vi "criticity safety.vi"() -> ()   [LabVIEW 2020]
uses:
  <vilib>/Utility/miscctls.llb/LVAnnotationListTypeDef.ctl
  <vilib>/Analysis/baseanly.llb/Mean (DBL).vi
  global/SettingVariable.vi
  <userlib>/_OpenG.lib/array/array.llb/Empty 2D Array (DBL)__ogtk.vi
  <vilib>/express/express arith-compare/Formula/XNode/ExpressFormulaBlockNode.xnode
  <vilib>/Analysis/NI_AALBase.lvlib
  <vilib>/Analysis/NI_AALPro.lvlib
panel:
  out "历史波形图":cluster{dbl, dbl, dbl[][]}(graph)
  out "左选标时刻":timestamp caption="左选标时刻：" format="%<%.2X %x>T"
  out "数据点数":i32 caption="选中的数据点数："
  out "通量通道均值":dbl
  out "临界途径均值":dbl
  in  "临界途径":u16(ring) caption="临界途径：" items=["棒位D"]
  in  "通量通道":u16(ring) caption="通量通道：" items=["电压8", "电流1", "电流2"]
  out "采样间隔":dbl
  out "开始时间":timestamp
  in  "在线数据":bool
  in  "打开文件":bool
  out "记录表":string[][](table) caption="计算结果记录表"
  out "临界外推趋势图":cluster{dbl[], dbl[]}[](graph) caption="XY Graph - Dark"
  in  "保存表格":bool
  in  "添加记录":bool
  out "提示信息":string="载入数据后，拖动波形图中的游标选取数据添加记录。"
  out "文件信息":string
  # "坐标轴与图例"
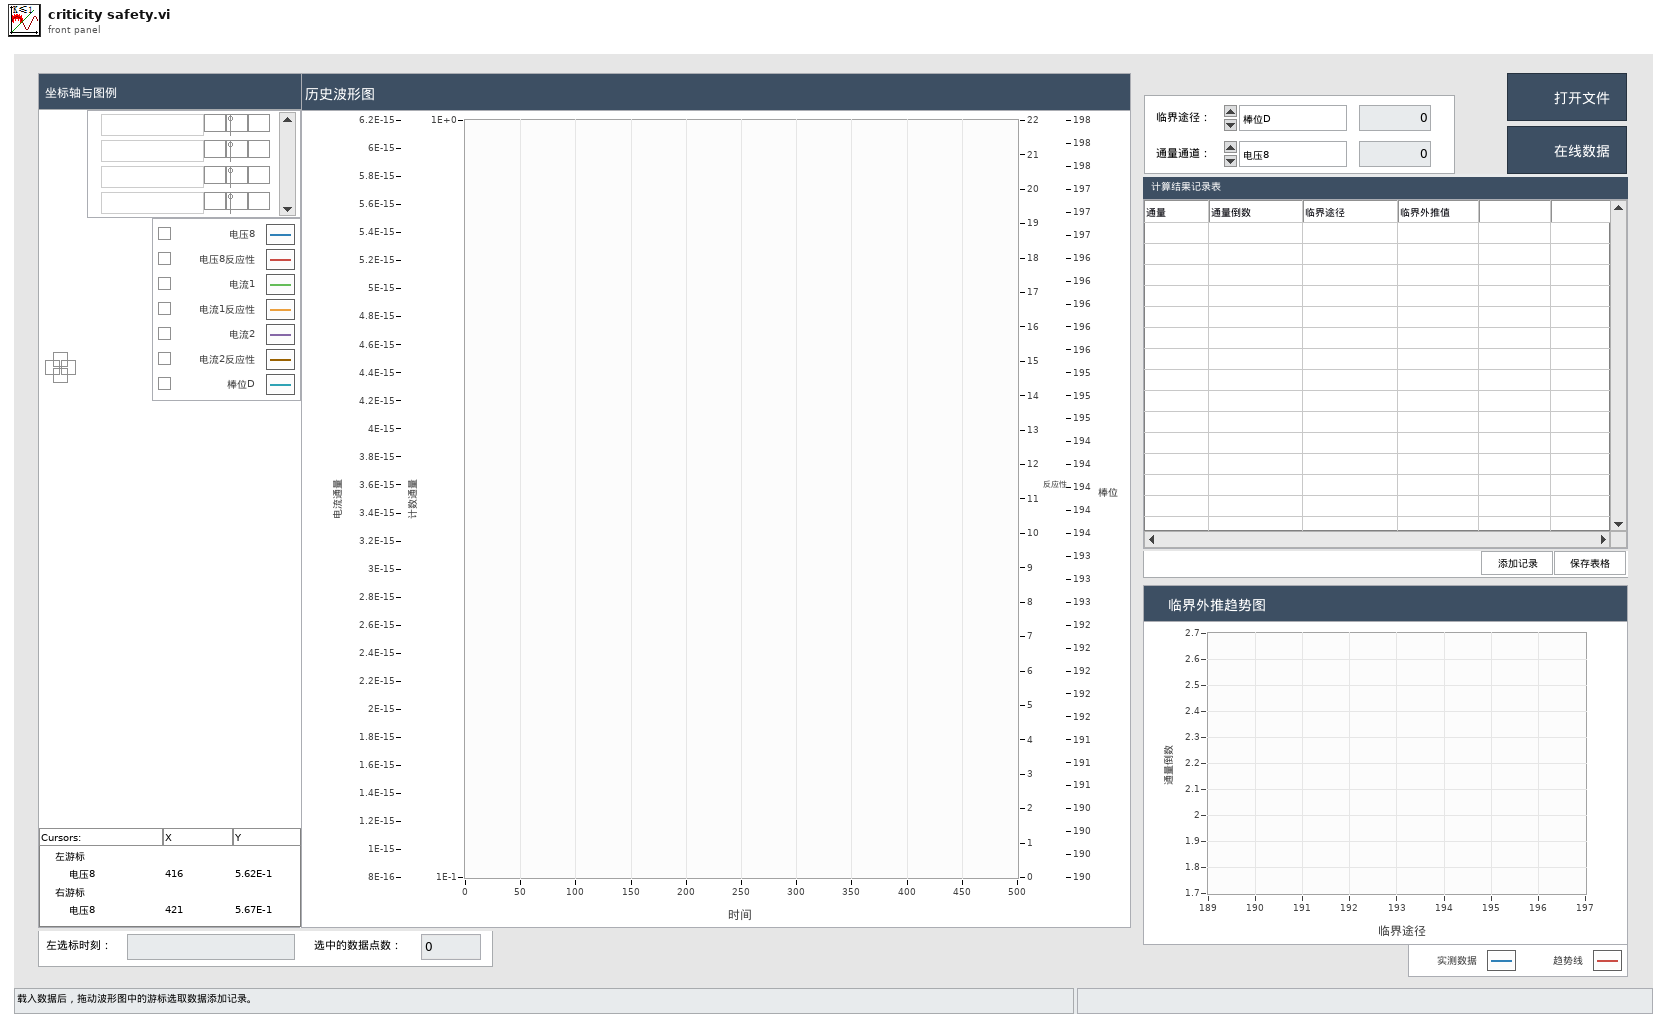
[diagram p1: front panel]
types:
  T1 = typedef "LVAnnotationListTypeDef.ctl" = cluster{"Name":string, "Color":u32, "Style":u8, "Point Style":u8, "Name Visible":bool, "Allow Drag":bool, "Annotation Mode":u32, "Plot":i32, "Index":i32, "Position":cluster{"X":dbl, "Y":dbl}, "X Scale":u32, "Y Scale":u32, "Show Arrow":bool, "Lock Name":bool, "Plot Area":i32, "Label Offset":cluster{"X":dbl, "Y":dbl}}[]
  T2 = cluster{"Name":string, "Color":u32, "Style":u8, "Point Style":u8, "Name Visible":bool, "Allow Drag":bool, "Annotation Mode":u32, "Plot":i32, "Index":i32, "Position":cluster{"X":dbl, "Y":dbl}, "X Scale":u32, "Y Scale":u32, "Show Arrow":bool, "Lock Name":bool, "Plot Area":i32, "Label Offset":cluster{"X":dbl, "Y":dbl}}
  T3 = enum16{"open", "replace", "create", "open or create", "replace or create", "replace or create with confirmation"}
  T4 = typedef "LVCursorListTypeDef.ctl" = cluster{"Name":string, "Color":u32, "Style":u8, "Point Style":u8, "Name Visible":bool, "Allow Drag":bool, "Cursor Mode":u32, "Plot":i32, "Index":i32, "Position":cluster{"X":dbl, "Y":dbl}, "X Scale":u32, "Y Scale":u32, "Watch Plots":i32[], "Watch All Plots":bool, "Plot Area":i32, "Label Offset":cluster{"X":dbl, "Y":dbl}}[]
  T5 = cluster{"Name":string, "Color":u32, "Style":u8, "Point Style":u8, "Name Visible":bool, "Allow Drag":bool, "Cursor Mode":u32, "Plot":i32, "Index":i32, "Position":cluster{"X":dbl, "Y":dbl}, "X Scale":u32, "Y Scale":u32, "Watch Plots":i32[], "Watch All Plots":bool, "Plot Area":i32, "Label Offset":cluster{"X":dbl, "Y":dbl}}
  T6 = enum32{"invalid app kind", "Development System", "Run Time System", "Student Edition", "Embedded LabVIEW", "Evaluation", "Custom"}
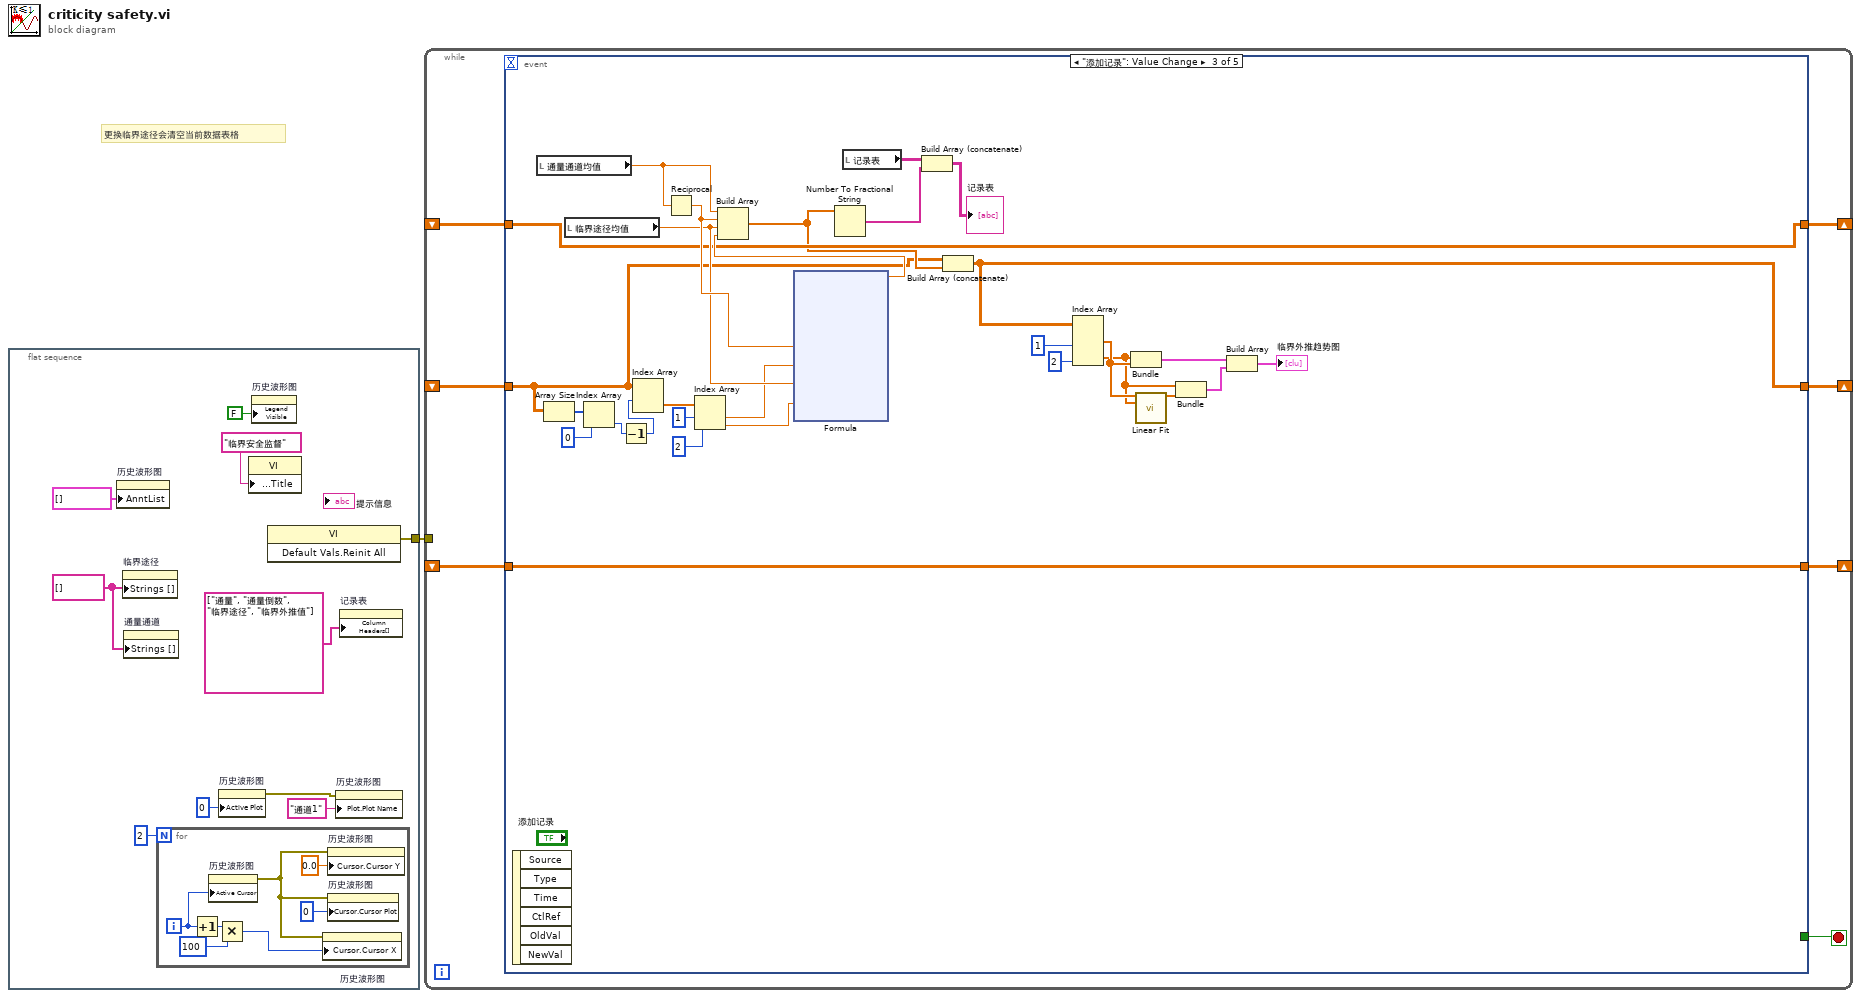
[diagram p0: block diagram]
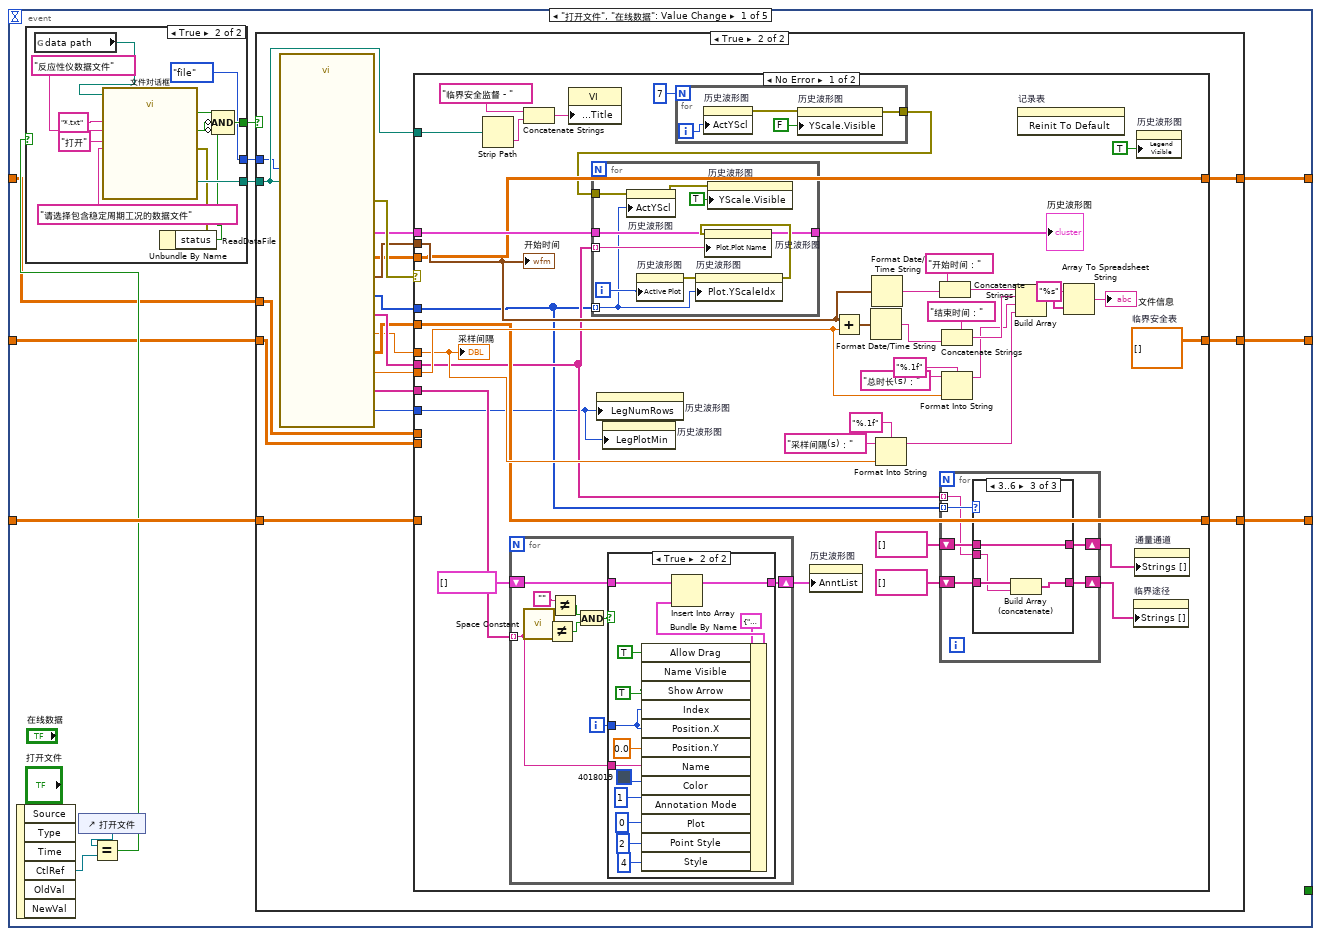
[diagram p2: hidden frame]
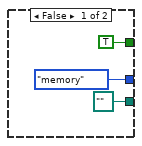
[diagram p3: hidden frame]
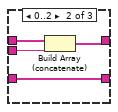
[diagram p6: hidden frame]
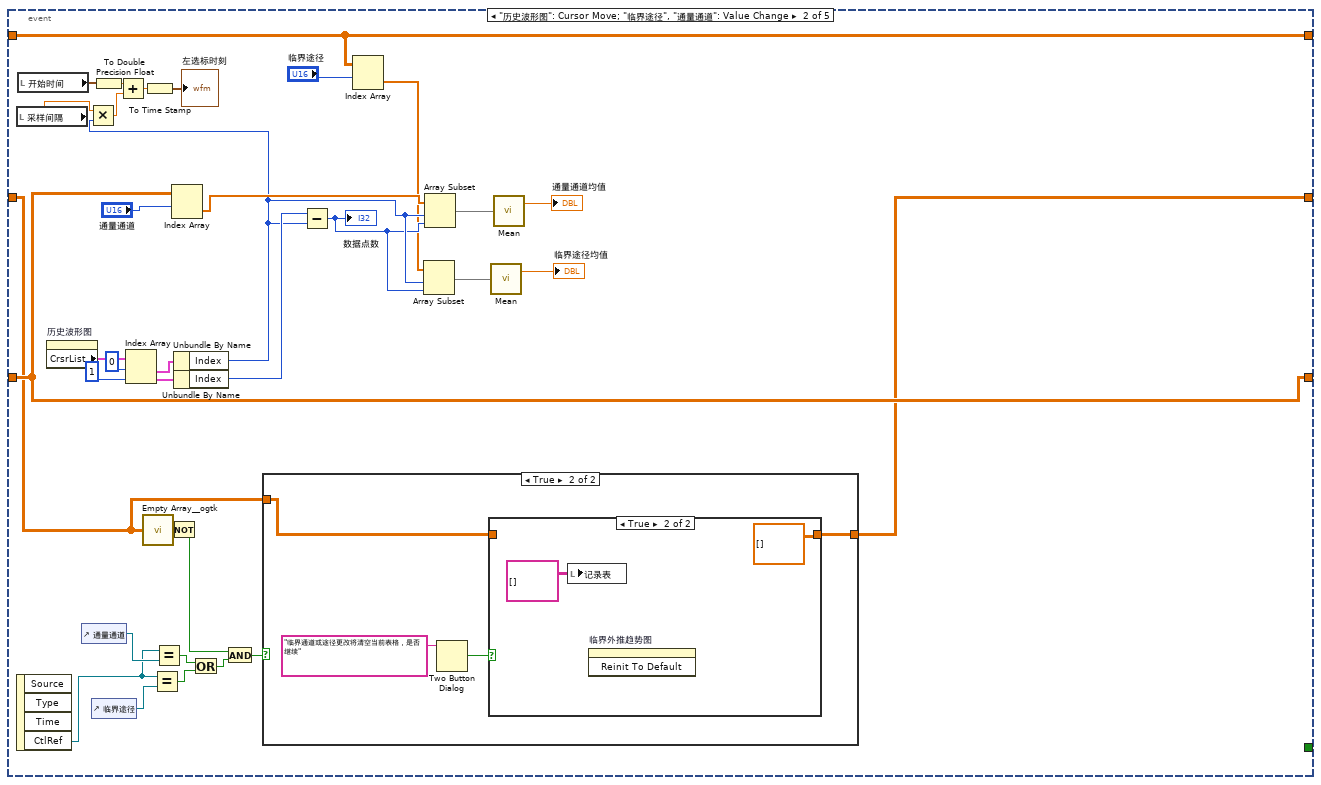
[diagram p9: hidden frame]
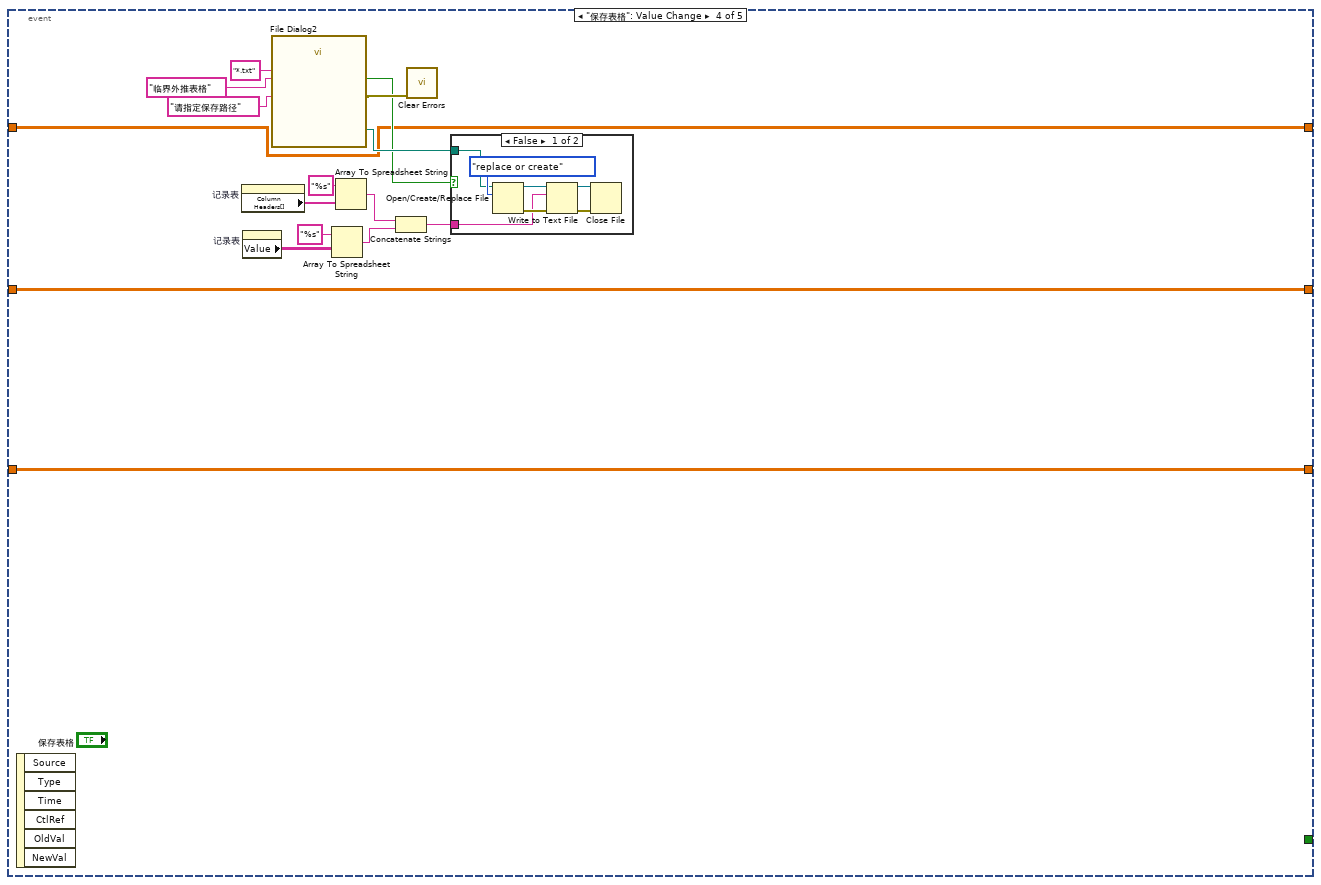
[diagram p12: hidden frame]
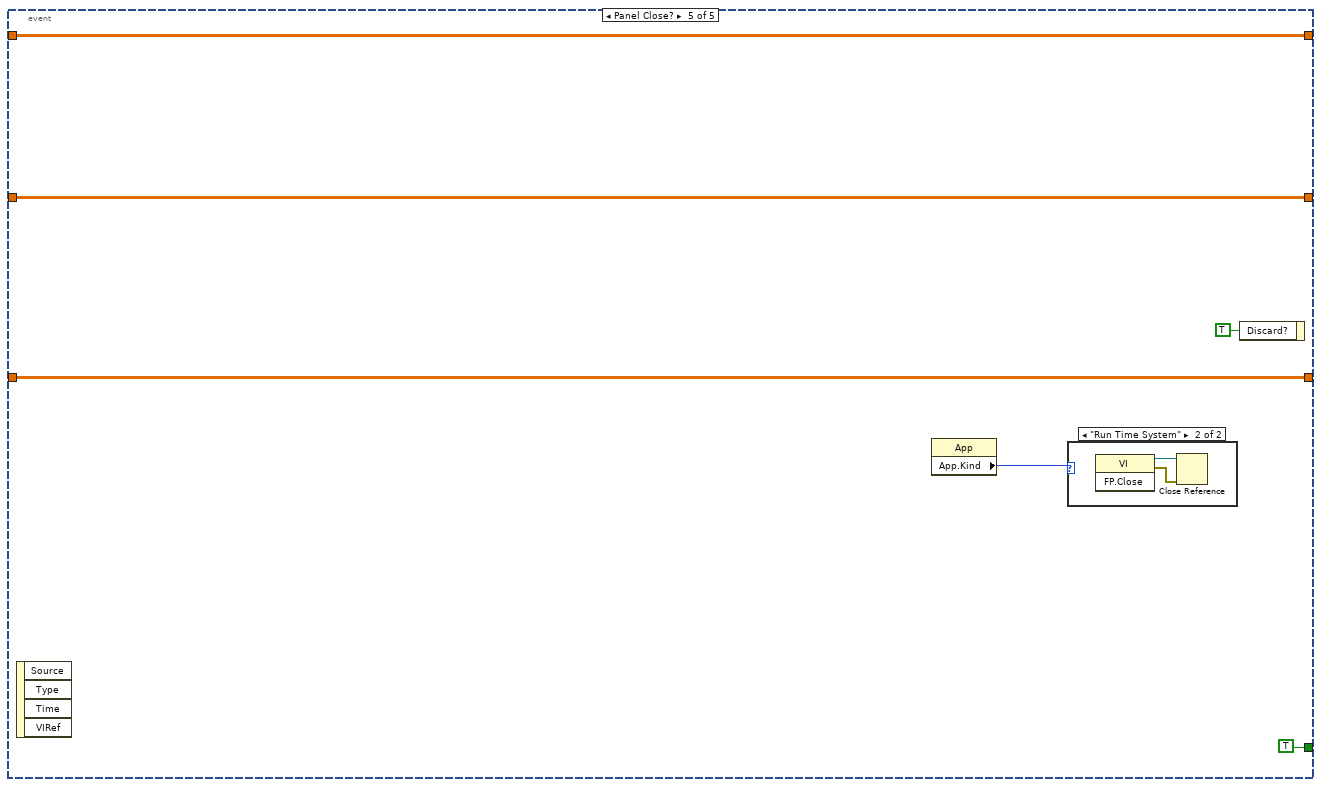
[diagram p14: hidden frame]
diagram:
  # "更换临界途径会清空当前数据表格"
  n1 = flat-sequence {
    tunnel: [w7] -> w1
    frame #0 {
      w2 = string[] [] ("Strings []")
      n2 = property on="历史波形图" class="WFGraph (strict)"("AnntList"=T1 [] ("Annotation List")) -> ()  [unwired: 2 in, 2 out]
      n3 = property on="临界途径" class="Ring (strict)"("Strings []"=w2) -> ()  [unwired: 2 in, 2 out]
      n4 = property on="通量通道" class="Ring (strict)"("Strings []"=w2) -> ()  [unwired: 2 in, 2 out]
      n5 = for {
        N: 2 -> [_]
        i -> [w16]
        n6 = Increment(x=w16) -> (x+1=w15:i32)
        n7 = property on="历史波形图" class="WFGraph (strict)"("Active Cursor"=w16) -> (error out=w12:errorcluster)  [unwired: 2 in, 1 out]
        n8 = Multiply(x=w15, y=100) -> (x*y=w13:i32)
        n9 = property on="历史波形图" class="WFGraph (strict)"(error in=w12, "Cursor.Cursor X"=w13) -> ()  [unwired: 1 in, 2 out]
        n10 = property on="历史波形图" class="WFGraph (strict)"(error in=w12, "Cursor.Cursor Y"=0.0 ("Cursor.Cursor Position:Cursor Y")) -> ()  [unwired: 1 in, 2 out]
        n11 = property on="历史波形图" class="WFGraph (strict)"(error in=w12, "Cursor.Cursor Plot"=0 ("Cursor.Cursor Index")) -> ()  [unwired: 1 in, 2 out]
      }
      n12 = property on="历史波形图" class="WFGraph (strict)"("Active Plot"=u32 0) -> (error out=w9:errorcluster)  [unwired: 2 in, 1 out]
      n13 = property class="VI"("Front Panel.Title"="临界安全监督" ("Front Panel Window:Title")) -> ()  [unwired: 2 in, 2 out]
      n14 = property on="历史波形图" class="WFGraph (strict)"("Legend Visible"=FALSE ("Legend:Visible")) -> ()  [unwired: 2 in, 2 out]
      n15 = invoke class="VI" method="Default Vals.Reinit All"() -> (error out=w7:errorcluster)  [unwired: 3 in, 2 out]
      n16 = property on="历史波形图" class="WFGraph (strict)"(error in=w9, "Plot.Plot Name"="通道1") -> ()  [unwired: 1 in, 2 out]
      n17 = property on="记录表" class="Tbl (strict)"("Column Headers[]"=string[] ["通量", "通量倒数", "临界途径", "临界外推值"] ("行首字符串[]")) -> ()  [unwired: 2 in, 2 out]
    }
  }
  n18 = while {
    shift-right: [w25] -> _
    shift-left: _ -> [w24]
    tunnel: w1 -> [_]
    shift-right: [w22] -> _
    shift-left: _ -> [w21]
    shift-right: [w19] -> _
    shift-left: _ -> [w20]
    stop <- w23 stop-if-true
    n19 = event shown="[2] \"添加记录\": Value Change" {
      selector: _ -> [_ _ _ _ _]
      dyn-events: _ -> [_ _ _ _ _]
      timeout: _ -> [_ _ _ _ _]
      tunnel: [w36 w184 w243 w273 w282] -> w25
      tunnel: w24 -> [w35 w184 w243 w273 w282]
      tunnel: [_ _ _ _ TRUE] -> w23
      tunnel: [w29 w183 w226 w259 w283] -> w22
      tunnel: w21 -> [w28 w183 w226 w259 w283]
      tunnel: w20 -> [w26 w173 w224 w258 w281]
      tunnel: [w27 w172 w223 w258 w281] -> w19
      event "打开文件", "在线数据": Value Change {
        n20 = event-data() -> ("CtlRef"=w33:refnum<vi>)  [unwired: 1 in, 5 out]
        n21 = control-ref of="打开文件"() -> (w32:refnum<vi>)
        n22 = Equal?(x=w32, y=w33) -> (x = y?=w31:bool)
        n23 = case shown="True" w31 {
          tunnel: [path "" ("selected path") w52] -> w37
          tunnel: [TRUE w43] -> w34
          tunnel: [enum16{"file", "memory"}."memory" ("source") enum16{"file", "memory"}."file" ("source")] -> w30
          frame False {
          }
          frame True {
            n24 = global read "SettingVariable.vi" "data path"() -> (w42:path)
            n25 = call "文件对话框"("start path"=w42, "prompt"="请选择包含稳定周期工况的数据文件", "button label"="打开", "pattern (all files)"="*.txt", "pattern label"="反应性仪数据文件") -> ("selected path"=w52:path, "exists"=w46:bool, "cancelled"=w45:bool, "error out"=w47:errorcluster)  [unwired: 7 in]
            n26 = Unbundle By Name(w47) -> ("status"=w44:bool)
            n27 = Compound Arithmetic op=AND(w46, invert w45, invert w44) -> (w43:bool)
          }
        }
        n28 = case shown="True" w34 {
          tunnel: w37 -> [_ w62]
          tunnel: [w55 w66] -> w36
          tunnel: w35 -> [w55 w65]
          tunnel: w30 -> [_ w61]
          tunnel: [w54 w59] -> w29
          tunnel: w28 -> [w54 w58]
          tunnel: [w53 w57] -> w27
          tunnel: w26 -> [w53 w56]
          frame False {
          }
          frame True {
            n29 = call "ReadDataFile.vi"("file path"=w62, "source"=w61) -> ("曲线对应标尺编号"=w69:i32[], "曲线名"=w68:string[], "通量数据"=w67:dbl[][], "时间间隔"=w64:dbl, "P2数据"=w60:dbl[][], "曲线数"=w71:i32, "开始时间"=w63:timestamp, "总时长(s)"=w72:dbl, "error out"=w74:errorcluster, "备注数组"=w70:string[], "波形簇"=w73:cluster{dbl, dbl, dbl[][]})  [unwired: 1 in, 2 out]
            n30 = case shown="No Error" w74 {
              tunnel: w73 -> [w87 _]
              tunnel: w72 -> [w106 _]
              tunnel: w71 -> [w75 _]
              tunnel: w70 -> [w113 _]
              tunnel: w69 -> [w78 _]
              tunnel: w68 -> [w83 _]
              tunnel: w67 -> [w84 _]
              tunnel: [w84 w171] -> w66
              tunnel: w65 -> [_ w171]
              tunnel: w64 -> [w104 _]
              tunnel: w63 -> [w111 _]
              tunnel: w62 -> [w90 _]
              tunnel: w60 -> [w86 _]
              tunnel: [w86 w170] -> w59
              tunnel: w58 -> [_ w170]
              tunnel: [w85 w169] -> w57
              tunnel: w56 -> [_ w169]
              frame No Error {
                w85 = dbl[][] []  # 临界安全表
                n31 = Strip Path(path=w90) -> (name=w91:string)  [unwired: 1 out]
                n32 = for {
                  tunnel: w113 -> [w148] mode=indexing
                  shift-right: [w150] -> w115
                  shift-left: T1 [] ("注释列表") -> [w151]
                  i -> [w152]
                  n33 = call <vilib>:"Space Constant.vi"() -> ("String"=w153:string)
                  n34 = Not Equal?(x=w153, y=w148) -> (x != y?=w146:bool)
                  n35 = Not Equal?(x="", y=w148) -> (x != y?=w147:bool)
                  n36 = And(x=w147, y=w146) -> (x .and. y?=w145:bool)
                  n37 = case shown="True" w145 {
                    tunnel: w148 -> [_ w163]
                    tunnel: w152 -> [_ w165]
                    tunnel: w151 -> [w154 w168]
                    tunnel: [w154 w167] -> w150
                    frame False {
                    }
                    frame True {
                      w166 = TRUE ("Show Arrow")
                      n38 = Bundle By Name(cluster=T2 {"Name"="", "Color"=0, "Style"=0, "Point Style"=0, "Name Visible"=FALSE, "Allow Drag"=FALSE, "Annotation Mode"=0, "Plot"=0, "Index"=0, "Position"={"X"=0.0, "Y"=0.0}, "X Scale"=0, "Y Scale"=0, "Show Arrow"=FALSE, "Lock Name"=FALSE, "Plot Area"=0, "Label Offset"={"X"=0.0, "Y"=0.0}} ("元素"), "Allow Drag"=TRUE, "Name Visible"=w166, "Show Arrow"=w166, "Index"=w165, "Position.X"=w165, "Position.Y"=0.0 ("Y"), "Name"=w163, "Color"=u32 4018019, "Annotation Mode"=u32 1, "Plot"=0, "Point Style"=u8 2, "Style"=u8 4) -> (w164:T2)
                      n39 = Insert Into Array(array=w168, new element=w164) -> (w167:T1)  [unwired: 1 in]
                    }
                  }
                }
                n40 = Concatenate Strings("临界安全监督 - " ("string"), w91) -> (w92:string)
                n41 = property class="VI"("Front Panel.Title"=w92) -> ()  [unwired: 2 in, 2 out]
                n42 = property on="历史波形图" class="WFGraph (strict)"("LegNumRows"=w75) -> ()  [unwired: 2 in, 2 out]
                n43 = property on="历史波形图" class="WFGraph (strict)"("LegPlotMin"=w75) -> ()  [unwired: 2 in, 2 out]
                n44 = for {
                  N: 7 -> [_]
                  tunnel: [w117] -> w76
                  i -> [w116]
                  n45 = property on="历史波形图" class="WFGraph (strict)"("ActYScl"=w116) -> (error out=w118:errorcluster)  [unwired: 2 in, 1 out]
                  n46 = property on="历史波形图" class="WFGraph (strict)"(error in=w118, "YScale.Visible"=FALSE ("Y Scale.Visible")) -> (error out=w117:errorcluster)  [unwired: 1 in, 1 out]
                }
                n47 = for {
                  tunnel: w78 -> [w139] mode=indexing
                  tunnel: w83 -> [w141] mode=indexing
                  tunnel: [w140] -> w88
                  tunnel: w87 -> [w140]
                  tunnel: w76 -> [w136]
                  i -> [w142]
                  n48 = property on="历史波形图" class="WFGraph (strict)"(error in=w136, "ActYScl"=w139) -> (error out=w137:errorcluster)  [unwired: 1 in, 1 out]
                  n49 = property on="历史波形图" class="WFGraph (strict)"("Active Plot"=w142) -> (error out=w144:errorcluster)  [unwired: 2 in, 1 out]
                  n50 = property on="历史波形图" class="WFGraph (strict)"(error in=w144, "Plot.YScaleIdx"=w139) -> (error out=w143:errorcluster)  [unwired: 1 in, 1 out]
                  n51 = property on="历史波形图" class="WFGraph (strict)"(error in=w143, "Plot.Plot Name"=w141) -> ()  [unwired: 1 in, 2 out]
                  n52 = property on="历史波形图" class="WFGraph (strict)"(error in=w137, "YScale.Visible"=TRUE ("Y Scale.Visible")) -> ()  [unwired: 1 in, 2 out]
                }
                "历史波形图" <- w88
                n53 = property on="历史波形图" class="WFGraph (strict)"("AnntList"=w115) -> ()  [unwired: 2 in, 2 out]
                n54 = Add(x=w111, y=w106) -> (x+y=w112:timestamp)
                n55 = Format Date/Time String(seconds (now)=w112) -> (date/time string=w107:string)  [unwired: 2 in]
                n56 = Format Date/Time String(seconds (now)=w111) -> (date/time string=w109:string)  [unwired: 2 in]
                n57 = Format Into String(format string="%.1f", initial string="采样间隔(s)：", w104) -> (resulting string=w97:string)  [unwired: 1 in, 1 out]
                n58 = Concatenate Strings("开始时间：" ("string"), w109) -> (w102:string)
                n59 = for {
                  tunnel: w83 -> [w120] mode=indexing
                  shift-right: [w121] -> w80
                  shift-left: string[] [] ("Strings []") -> [w122]
                  shift-right: [w123] -> w79
                  shift-left: string[] [] ("Strings []") -> [w124]
                  tunnel: w78 -> [w125] mode=indexing
                  n60 = case shown="3..6" w125 {
                    tunnel: w124 -> [w127 w131 w135]
                    tunnel: [w127 w130 w135] -> w123
                    tunnel: w122 -> [w126 w128 w134]
                    tunnel: [w126 w128 w132] -> w121
                    tunnel: w120 -> [_ w129 w133]
                    frame 7, Default {
                    }
                    frame 0..2 {
                      n61 = Build Array (concatenate)(w131, w129) -> (w130:string[])
                    }
                    frame 3..6 {
                      n62 = Build Array (concatenate)(w134, w133) -> (w132:string[])
                    }
                  }
                }
                n63 = Concatenate Strings("结束时间：" ("string"), w107) -> (w99:string)
                n64 = Format Into String(format string="%.1f", initial string="总时长(s)：", w106) -> (resulting string=w98:string)  [unwired: 1 in, 1 out]
                n65 = Build Array(w102, w99, w98, w97) -> (w101:string[])
                n66 = invoke on="记录表" class="Tbl (strict)" method="Reinit To Default"() -> ()  [unwired: 3 in, 3 out]
                n67 = Array To Spreadsheet String(array=w101, 3:"%s" ("format string")) -> (spreadsheet string=→"文件信息":string)  [unwired: 1 in]
                n68 = property on="临界途径" class="Ring (strict)"("Strings []"=w80) -> ()  [unwired: 2 in, 2 out]
                n69 = property on="通量通道" class="Ring (strict)"("Strings []"=w79) -> ()  [unwired: 2 in, 2 out]
                n70 = property on="历史波形图" class="WFGraph (strict)"("Legend Visible"=TRUE ("Legend:Visible")) -> ()  [unwired: 2 in, 2 out]
                "开始时间" <- w111
                "采样间隔" <- w104
              }
              frame Error {
              }
            }
          }
        }
      }
      event "历史波形图": Cursor Move; "临界途径", "通量通道": Value Change {
        n71 = local read "采样间隔"() -> (w195:dbl)
        n72 = event-data() -> ("CtlRef"=w180:refnum<vi>)  [unwired: 1 in, 3 out]
        n73 = local read "开始时间"() -> (w196:timestamp)
        n74 = property on="历史波形图" class="WFGraph (strict)"() -> ("CrsrList"=w202:T4)  [unwired: 2 in, 2 out]
        n75 = control-ref of="通量通道"() -> (w181:refnum<vi>)
        n76 = control-ref of="临界途径"() -> (w182:refnum<vi>)
        n77 = To Double Precision Float(number=w196) -> (double precision float=w201:dbl)
        n78 = Index Array(array=w202, index #1=0 ("index"), index #2=1 ("index")) -> (element #1=w204:T5, element #2=w206:T5)
        n79 = call-poly <userlib>:"Empty Array__ogtk.vi"("Array"=w173) -> ("Empty Array?"=w177:bool)  [unwired: 8 in]
        n80 = Equal?(x=w180, y=w182) -> (x = y?=w178:bool)
        n81 = Equal?(x=w180, y=w181) -> (x = y?=w179:bool)
        n82 = Not(x=w177) -> (.not. x?=w176:bool)
        n83 = Index Array(array=w184, index (row)="通量通道") -> (element=w192:dbl[])  [unwired: 1 in]
        n84 = Unbundle By Name(w204) -> ("Index"=w188:i32)
        n85 = Multiply(x=w195, y=w188) -> (x*y=w198:dbl)
        n86 = Add(x=w201, y=w198) -> (x+y=w200:dbl)
        n87 = To Time Stamp(1:w200) -> (0:→"左选标时刻":timestamp)
        n88 = Unbundle By Name(w206) -> ("Index"=w197:i32)
        n89 = Or(x=w179, y=w178) -> (x .or. y?=w175:bool)
        n90 = And(x=w176, y=w175) -> (x .and. y?=w174:bool)
        n91 = case shown="True" w174 {
          tunnel: w173 -> [w207 w209]
          tunnel: [w207 w208] -> w172
          frame False {
          }
          frame True {
            n92 = Two Button Dialog(message="临界通道或途径更改将清空当前表格，是否继续") -> (T button?=w211:bool)  [unwired: 2 in]
            n93 = case shown="True" w211 {
              tunnel: w209 -> [w212 _]
              tunnel: [w212 dbl[][] [] ("临界安全表")] -> w208
              frame False {
              }
              frame True {
                n94 = local write "记录表"(string[][] [] ("记录表")) -> ()
                n95 = invoke on="临界外推趋势图" class="XYGraph (strict)" method="Reinit To Default"() -> ()  [unwired: 3 in, 3 out]
              }
            }
          }
        }
        n96 = Subtract(x=w197, y=w188) -> (x-y=w187:i32)
        "数据点数" <- w187
        n97 = Index Array(array=w183, index (row)="临界途径") -> (element=w186:dbl[])  [unwired: 1 in]
        n98 = Array Subset(array=w186, index=w188, length=w187) -> (w185:dbl[])
        n99 = Array Subset(array=w192, index=w188, length=w187) -> (w194:dbl[])
        n100 = call-poly <vilib>:"Mean.vi"("X"=w185) -> ("mean"=→"临界途径均值":dbl)  [unwired: 1 out]
        n101 = call-poly <vilib>:"Mean.vi"("X"=w194) -> ("mean"=→"通量通道均值":dbl)  [unwired: 1 out]
      }
      event "添加记录": Value Change {
        n102 = event-data() -> ()  [unwired: 1 in, 6 out]
        n103 = local read "通量通道均值"() -> (w240:dbl)
        n104 = Array Size(array=w224) -> (size(s)=w235:i32[])
        n105 = local read "临界途径均值"() -> (w230:dbl)
        n106 = Index Array(array=w235, index=0) -> (element=w233:i32)
        n107 = Decrement(x=w233) -> (x-1=w232:i32)
        n108 = Index Array(array=w224, index (row)=w232) -> (element=w238:dbl[])  [unwired: 1 in]
        n109 = Reciprocal(x=w240) -> (1/x=w231:dbl)
        n110 = Index Array(array=w238, index #1=1 ("index"), index #2=2 ("index")) -> (element #1=w229:dbl, element #2=w228:dbl)
        n111 = xnode "Formula"("M1"=w231, "M2"=w229, "X1"=w230, "X2"=w228) -> ("Result"=w227:dbl)  [unwired: 1 in, 1 out]
        n112 = Build Array(w240, w231, w230, w227) -> (w225:dbl[])
        n113 = Number To Fractional String(number=w225) -> (F-format string=w239:string[])  [unwired: 3 in]
        n114 = local read "记录表"() -> (w242:string[][])
        n115 = Build Array (concatenate)(w242, w239) -> (→"记录表":string[][])
        n116 = Build Array (concatenate)(w224, w225) -> (w223:dbl[][])
        n117 = Index Array(array=w223, index (col) #1=1 ("index"), index (col) #2=2 ("index")) -> (element #1=w218:dbl[], element #2=w216:dbl[])  [unwired: 2 in]
        n118 = Bundle(w216, w218) -> (w220:cluster{dbl[], dbl[]})  [unwired: 1 in]
        n119 = call <vilib>:"Linear Fit.vi"("Y"=w218, "X"=w216) -> ("Best Linear Fit"=w217:dbl[])  [unwired: 9 in, 4 out]
        n120 = Bundle(w216, "Best Linear Fit"=w217) -> (w215:cluster{dbl[], "Best Linear Fit":dbl[]})  [unwired: 1 in]
        n121 = Build Array(w220, w215) -> (→"临界外推趋势图":cluster{dbl[], "Best Linear Fit":dbl[]}[])
      }
      event "保存表格": Value Change {
        n122 = event-data() -> ()  [unwired: 1 in, 6 out]
        n123 = property on="记录表" class="Tbl (strict)"() -> ("Column Headers[]"=w272:string[])  [unwired: 2 in, 2 out]
        n124 = property on="记录表" class="Tbl (strict)"() -> ("Value"=w269:string[][])  [unwired: 2 in, 2 out]
        n125 = call "File Dialog2"("prompt"="请指定保存路径" ("提示"), "pattern (all files)"="*.txt" ("类型（所有文件）"), "pattern label"="临界外推表格" ("默认名称")) -> ("selected path"=w266:path, "cancelled"=w265:bool, "error out"=w267:errorcluster)  [unwired: 9 in, 1 out]
        n126 = Array To Spreadsheet String(array=w269, 3:"%s" ("format string")) -> (spreadsheet string=w268:string)  [unwired: 1 in]
        n127 = Array To Spreadsheet String(array=w272, 3:"%s" ("格式字符串")) -> (spreadsheet string=w271:string)  [unwired: 1 in]
        n128 = Concatenate Strings(w271, w268) -> (w270:string)
        n129 = call <vilib>:"Clear Errors.vi"("error in (no error)"=w267) -> ()  [unwired: 5 in, 2 out]
        n130 = case shown="False" w265 {
          tunnel: w270 -> [w275 _]
          tunnel: w266 -> [w274 _]
          frame False {
            n131 = Open/Create/Replace File(file path (use dialog)=w274, operation (0:open)=T3."replace or create") -> (refnum out=w278:refnum<file>, error out=w280:errorcluster)  [unwired: 4 in, 1 out]
            n132 = Write to Text File(file (use dialog)=w278, text=w275, error in=w280) -> (refnum out=w277:refnum<file>, error out=w276:errorcluster)  [unwired: 1 in, 1 out]
            n133 = Close File(refnum=w277, error in=w276) -> ()  [unwired: 2 out]
          }
          frame True {
          }
        }
      }
      event Panel Close? {
        n134 = event-data() -> ()  [unwired: 1 in, 4 out]
        n135 = property class="App"() -> ("App.Kind"=w284:T6)  [unwired: 2 in, 2 out]
        n136 = case shown="\"Run Time System\"" w284 {
          frame "Development System", Default {
          }
          frame "Run Time System" {
            n137 = invoke class="VI" method="FP.Close"() -> (reference out=w287:refnum<vi>, error out=w288:errorcluster)  [unwired: 3 in, 1 out]
            n138 = Close Reference(reference=w287, error in (no error)=w288) -> ()  [unwired: 1 out]
          }
        }
        n139 = event-data("Discard?"=TRUE) -> ()  [unwired: 1 in, 1 out]
      }
    }
  }
